vi "Global IO.vi"() -> ()   [LabVIEW 2011]
panel:
  in  "DO":bool[](array[boolean])
  out "DI":bool[](array[boolean])
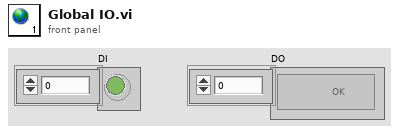
[diagram p1: front panel]
diagram:
